vi "Error Data.vi"(8 "error in (no error)":errorcluster, 10 "error input":errorcluster, 11 "Debug UI in":refnum<class "Debug UI.lvclass">) -> (0 "error out":errorcluster, 3 "Debug UI out":refnum<class "Debug UI.lvclass">)   [LabVIEW 2016, in "Assert API Components.lvlib" / "Log Assert Core.lvlib" / "Debug UI.lvclass"]
uses:
  Debug UI.lvclass
  Debug UI.lvclass/Debug UI.ctl
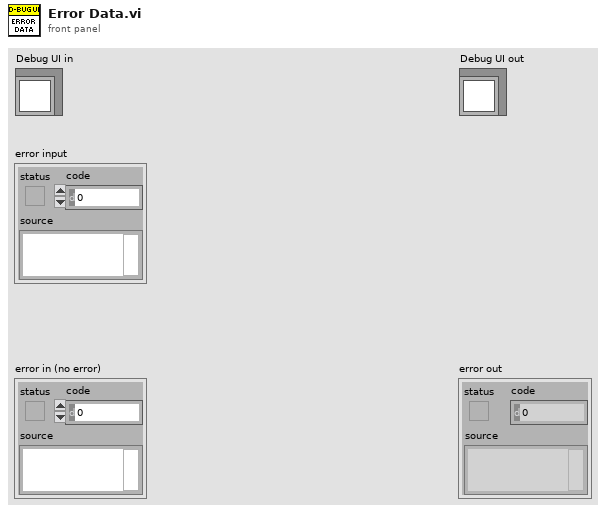
[diagram p1: front panel]
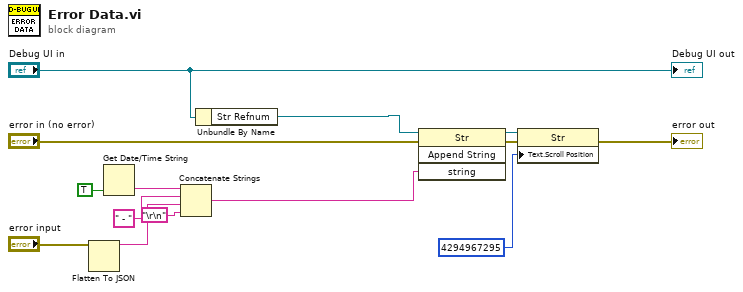
[diagram p0: block diagram]
diagram:
  n1 = Flatten To JSON(anything="error input") -> (JSON string=w8:string)  [unwired: 2 in, 1 out]
  n2 = Get Date/Time String(want seconds? (F)=TRUE) -> (time string=w10:string)  [unwired: 2 in, 1 out]
  n3 = Concatenate Strings(w10, " - " ("string"), w8, "\r\n") -> (w4:string)
  n4 = Unbundle By Name("Debug UI in") -> ("Str Refnum"=w12:refnum<vi>)
  n5 = invoke class="Str" method="Append String"(reference=w12, error in="error in (no error)", "string"=w4) -> (reference out=w3:refnum<vi>, error out=w2:errorcluster)  [unwired: 1 in, 2 out]
  n6 = property class="Str"(reference=w3, error in=w2, "Text.Scroll Position"=u32 4294967295) -> (error out=→"error out":errorcluster)  [unwired: 1 out]
  "Debug UI out" <- "Debug UI in"
